vi "小数位数写入.vi"(4 "error in (no error)":errorcluster caption="错误输入（无错误）", 5 "Value":u8 caption="值", 6 "Container State":T2 caption="容器状态", 7 "Display State In":T1={"显示位数"=6, "小数位数"=0} caption="显示状态输入") -> (0 "error out":errorcluster caption="错误输出", 3 "Display State Out":T1={"显示位数"=6, "小数位数"=0} caption="显示状态输出")   [LabVIEW 2013, in "数码管.xctl"]
uses:
  <vilib>/_xctls/Container State.ctl
  <vilib>/_xctls/XControlSupport.lvlib
panel:
  # "将以下值显示控件替换为所需类型的显示控件。\n不要从连线板中删除该显示控件或其它显示控件。\n不要更改连线板模式。\n值显示控件应始终位于连线板输出端自顶部起第三个接线端。"
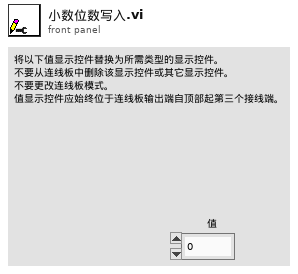
[diagram p1: front panel]
types:
  T1 = typedef "数码管.xctl/数码管.ctl" = cluster{"显示位数":u8, "小数位数":u8}
  T2 = typedef "XControlSupport.lvlib/Container State.ctl" = cluster{"Indicator?":bool, "Run Mode?":bool, " Refnum":refnum<vi>}
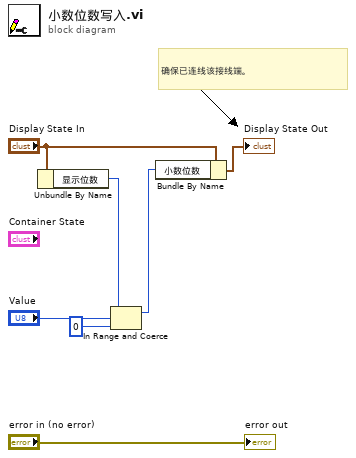
[diagram p0: block diagram]
diagram:
  # "确保已连线该接线端。"
  n1 = Unbundle By Name("Display State In") -> ("显示位数"=w2:u8)
  n2 = In Range and Coerce(upper limit=w2, x="Value", lower limit=u8 0 ("下限")) -> (coerced(x)=w1:u8)  [unwired: 1 out]
  n3 = Bundle By Name(cluster="Display State In", "小数位数"=w1) -> (→"Display State Out":T1)
  "error out" <- "error in (no error)"
